vi "Test add points.vi"() -> ()   [LabVIEW 2019]
uses:
  Ctrl/cmd_common.ctl
panel:
  in  "tap":enum32{"Main", "Data"}(tab)
  out "Potential graph":dbl[][](graph)
  in  "Run":bool
  in  "clear":bool
  out "N of obstacles":i32(slide) scale=0.0..20.0
  in  "add obstacle":bool
  in  "Finish":bool
  out "Waypoint":cluster{"add arr":cluster{i32, i32}[]}[](graph)
  in  "global-val":T1={"KP"=5.0, "ETA"=100.0, "AREA_WIDTH"=30.0, "Osc_Det_Len"=3}
  in  "set-val":T2={"start pt"={"x"=0, "y"=10}, "goal pt"={"x"=30, "y"=30}, "grid size"=0.5, "robot radius"=5.0, "obstacles"=[{"x"=15, "y"=25}, {"x"=5, "y"=15}, {"x"=20, "y"=26}, {"x"=25, "y"=25}]}
  in  "add arr":cluster{i32, i32}[](array[cluster])
  out "add point":cluster{i32, i32}
  # "Made by Ybbaek"
  # "Potential Field Simulation"
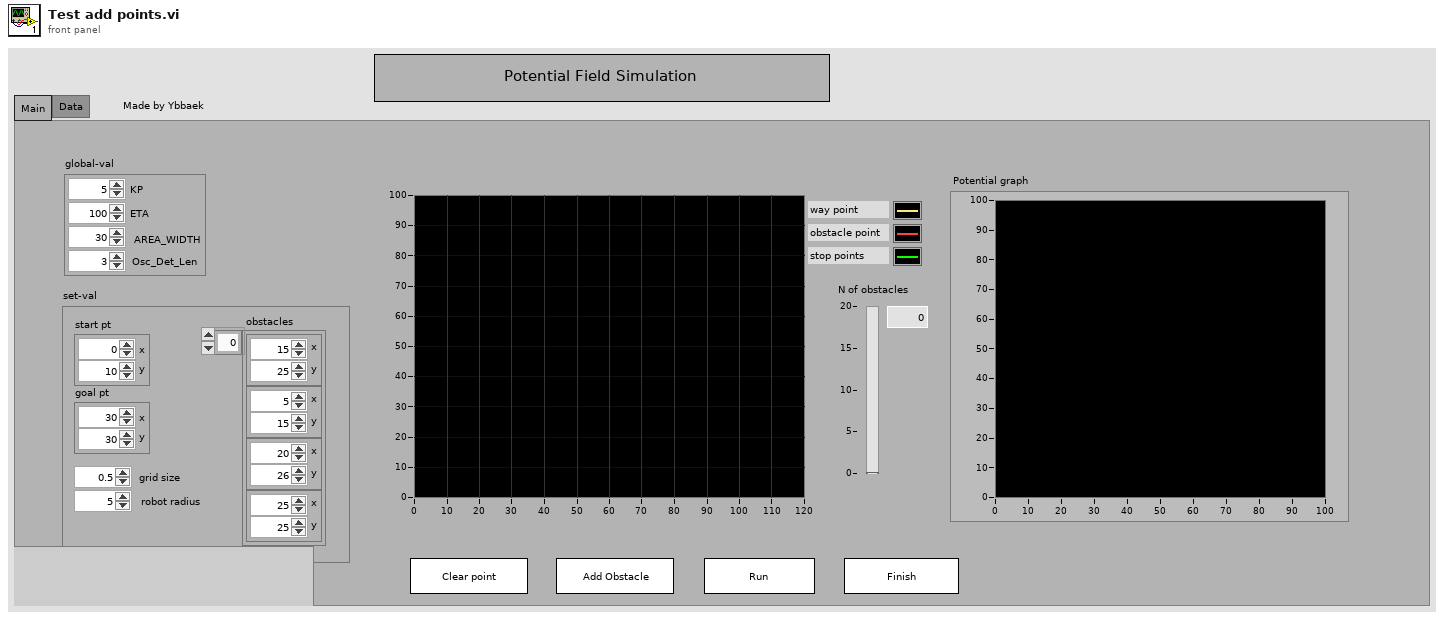
[diagram p1: front panel]
types:
  T1 = cluster{"KP":dbl, "ETA":dbl, "AREA_WIDTH":dbl, "Osc_Det_Len":u32}
  T2 = cluster{"start pt":cluster{"x":i32, "y":i32}, "goal pt":cluster{"x":i32, "y":i32}, "grid size":dbl, "robot radius":dbl, "obstacles":cluster{"x":i32, "y":i32}[]}
  T3 = typedef "cmd_common.ctl" = enum16{"read", "write"}
  T4 = typedef "LVPoint32TypeDef.ctl" = cluster{"Horizontal":i32, "Vertical":i32}
  T5 = typedef "LVRectTypeDef.ctl" = cluster{"Left":i16, "Top":i16, "Right":i16, "Bottom":i16}
  T6 = typedef "NI_Matrix.lvlib/RealMatrix.ctl" = dbl[][]
  T7 = cluster{"delay":dbl, "d":dbl, "rxy":cluster{"x":dbl, "y":dbl}[], "pmap":T6}
  T8 = cluster{"start pt":cluster{"x":i32, "y":dbl}, "goal pt":cluster{"x":dbl, "y":dbl}, "grid size":dbl, "robot radius":dbl, "obstacles":cluster{"x":i32, "y":i32}[]}
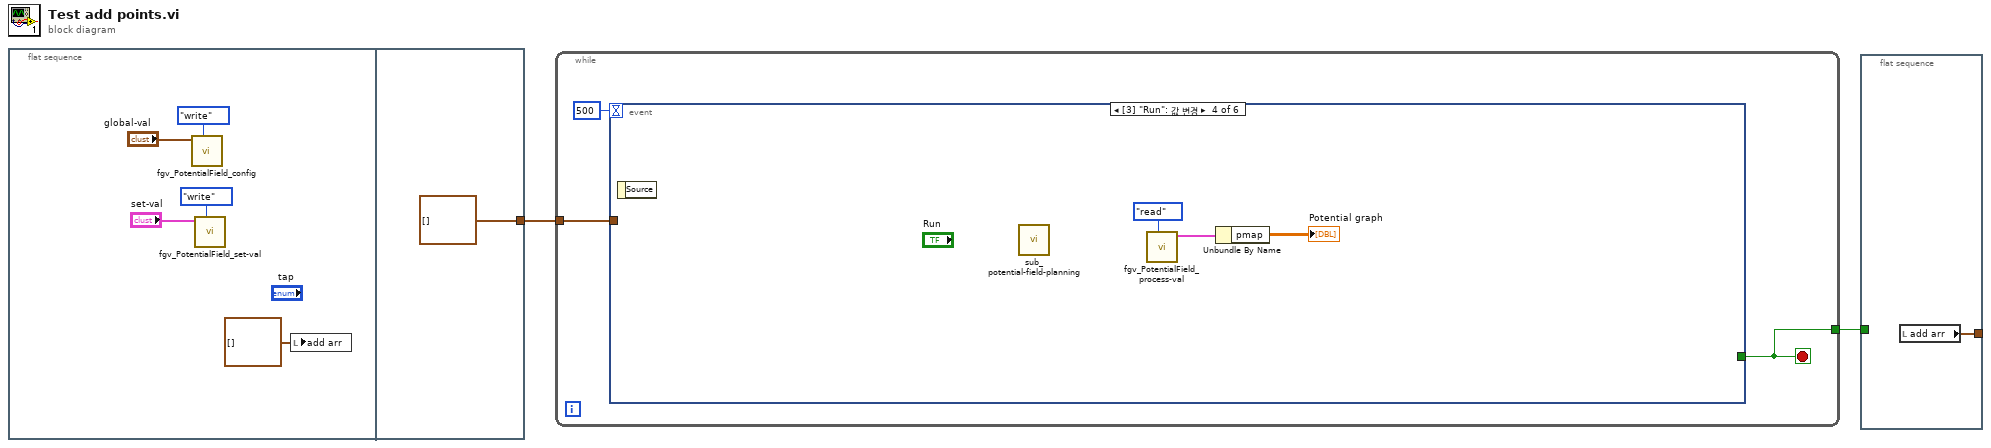
[diagram p0: block diagram]
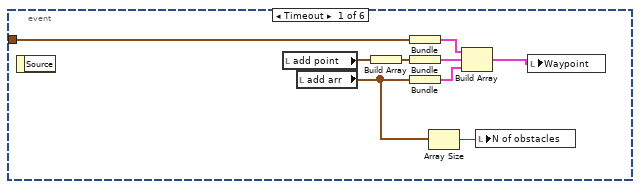
[diagram p2: hidden frame]
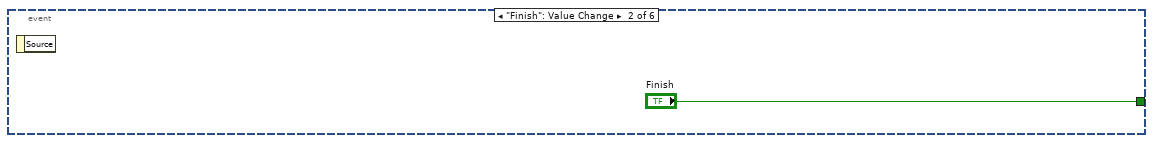
[diagram p3: hidden frame]
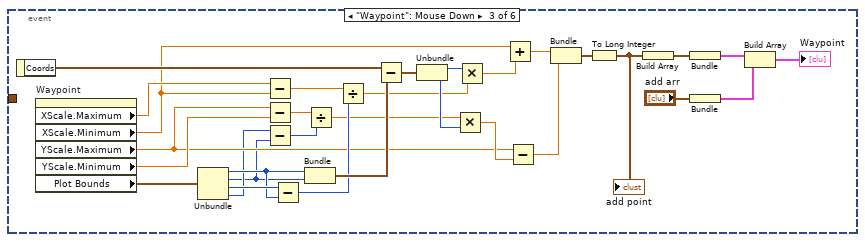
[diagram p4: hidden frame]
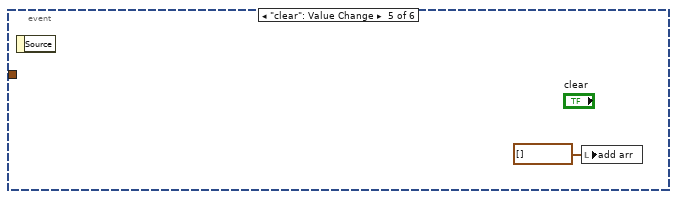
[diagram p5: hidden frame]
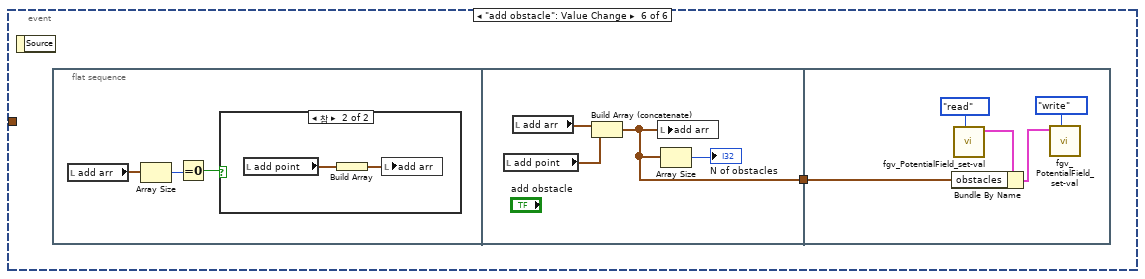
[diagram p6: hidden frame]
diagram:
  n1 = flat-sequence {
    tunnel: [cluster{"X":i32, "Y":i32}[] []] -> w1
    frame #0 {
      n2 = call "fgv_PotentialField_config.vi"("cmd"=cmd_common."write", "pf-val"="global-val") -> ()  [unwired: 9 in, 1 out]
      n3 = call "fgv_PotentialField_set-val.vi"("cmd"=cmd_common."write", "set-val"="set-val") -> ()  [unwired: 9 in, 1 out]
      n4 = local write "add arr"(cluster{i32, i32}[] [] ("add arr")) -> ()
    }
    frame #1 {
    }
  }
  n5 = while {
    tunnel: [w11] -> w2
    tunnel: w1 -> [w10]
    stop <- w11 stop-if-true
    n6 = event shown="[3] \"Run\": 값 변경" {
      selector: _ -> [_ _ _ _ _ _]
      dyn-events: _ -> [_ _ _ _ _ _]
      timeout: 500 -> [_ _ _ _ _ _]
      tunnel: [_ "Finish" _ _ _ _] -> w11
      tunnel: w10 -> [w14 _ _ _ _ _]
      event Timeout {
        n7 = event-data() -> ()  [unwired: 1 in, 1 out]
        n8 = local read "add point"() -> (w19:cluster{i32, i32})
        n9 = local read "add arr"() -> (w12:cluster{i32, i32}[])
        n10 = Build Array(w19) -> (w20:cluster{i32, i32}[])
        n11 = Bundle(w14) -> (w15:cluster{cluster{"X":i32, "Y":i32}[]})  [unwired: 1 in]
        n12 = Bundle(w20) -> (w18:cluster{cluster{i32, i32}[]})  [unwired: 1 in]
        n13 = Bundle("add arr"=w12) -> (w17:cluster{"add arr":cluster{i32, i32}[]})  [unwired: 1 in]
        n14 = Array Size(array=w12) -> (size(s)=w13:i32)
        n15 = Build Array(w15, w18, w17) -> (w16:cluster{"add arr":cluster{"X":i32, "Y":i32}[]}[])
        n16 = local write "N of obstacles"(w13) -> ()
        n17 = local write "Waypoint"(w16) -> ()
      }
      event "Finish": Value Change {
        n18 = event-data() -> ()  [unwired: 1 in, 1 out]
      }
      event "Waypoint": Mouse Down {
        n19 = event-data() -> ("Coords"=w51:T4)  [unwired: 1 in]
        n20 = property on="Waypoint" class="XYGraph (엄격한)"() -> ("XScale.Maximum"=w47:dbl, "XScale.Minimum"=w39:dbl, "YScale.Maximum"=w31:dbl, "YScale.Minimum"=w34:dbl, "Plot Bounds"=w52:T5)  [unwired: 2 in, 2 out]
        n21 = Unbundle(w52) -> ("Left"=w43:i16, "Top"=w29:i16, "Right"=w44:i16, "Bottom"=w30:i16)
        n22 = Subtract(x=w47, y=w39) -> (x-y=w42:dbl)
        n23 = Subtract(x=w31, y=w34) -> (x-y=w37:dbl)
        n24 = Subtract(x=w30, y=w29) -> (x-y=w36:i16)
        n25 = Subtract(x=w44, y=w43) -> (x-y=w41:i16)
        n26 = Bundle("Left"=w43, "Top"=w29) -> (w50:cluster{"Left":i16, "Top":i16})  [unwired: 1 in]
        n27 = Divide(x=w37, y=w36) -> (x/y=w35:dbl)
        n28 = Divide(x=w42, y=w41) -> (x/y=w24:dbl)
        n29 = Subtract(x=w51, y=w50) -> (x-y=w46:T4)
        n30 = Unbundle(w46) -> ("Horizontal"=w25:i32, "Vertical"=w45:i32)
        n31 = Multiply(x=w35, y=w45) -> (x*y=w33:dbl)
        n32 = Multiply(x=w25, y=w24) -> (x*y=w40:dbl)
        n33 = Add(x=w39, y=w40) -> (x+y=w38:dbl)
        n34 = Subtract(x=w31, y=w33) -> (x-y=w32:dbl)
        n35 = Bundle(w38, w32) -> (w23:cluster{dbl, dbl})  [unwired: 1 in]
        n36 = To Long Integer(number=w23) -> (32bit integer=w22:cluster{i32, i32})
        "add point" <- w22
        n37 = Build Array(w22) -> (w48:cluster{i32, i32}[])
        n38 = Bundle(w48) -> (w49:cluster{cluster{i32, i32}[]})  [unwired: 1 in]
        n39 = Bundle("add arr"="add arr") -> (w27:cluster{"add arr":cluster{i32, i32}[]})  [unwired: 1 in]
        n40 = Build Array(w49, w27) -> (→"Waypoint":cluster{"add arr":cluster{i32, i32}[]}[])
      }
      event "Run": Value Change {
        n41 = event-data() -> ()  [unwired: 1 in, 1 out]
        n42 = call "sub_potential-field-planning.vi"() -> ()  [unwired: 12 in]
        n43 = call "fgv_PotentialField_process-val.vi"("cmd"=cmd_common."read") -> ("prcess val out"=w54:T7)  [unwired: 10 in]
        n44 = Unbundle By Name(w54) -> ("pmap"=→"Potential graph":T6)
      }
      event "clear": Value Change {
        n45 = event-data() -> ()  [unwired: 1 in, 1 out]
        n46 = local write "add arr"(cluster{dbl, dbl}[] [] ("add arr")) -> ()
      }
      event "add obstacle": Value Change {
        n47 = event-data() -> ()  [unwired: 1 in, 1 out]
        n48 = flat-sequence {
          tunnel: [w63] -> w57
          tunnel: w57 -> [w67]
          frame #0 {
            n49 = local read "add arr"() -> (w60:cluster{i32, i32}[])
            n50 = Array Size(array=w60) -> (size(s)=w59:i32)
            n51 = Equal To 0?(x=w59) -> (x = 0?=w58:bool)
            n52 = case shown="참" w58 {
              frame False {
              }
              frame True {
                n53 = local read "add point"() -> (w62:cluster{i32, i32})
                n54 = Build Array(w62) -> (w61:cluster{i32, i32}[])
                n55 = local write "add arr"(w61) -> ()
              }
            }
          }
          frame #1 {
            n56 = local read "add point"() -> (w65:cluster{i32, i32})
            n57 = local read "add arr"() -> (w66:cluster{i32, i32}[])
            n58 = Build Array (concatenate)(w66, w65) -> (w63:cluster{i32, i32}[])
            n59 = local write "add arr"(w63) -> ()
            n60 = Array Size(array=w63) -> (size(s)=→"N of obstacles":i32)
          }
          frame #2 {
            n61 = call "fgv_PotentialField_set-val.vi"("cmd"=cmd_common."read") -> ("set-val out"=w69:T8)  [unwired: 10 in]
            n62 = Bundle By Name(cluster=w69, "obstacles"=w67) -> (w68:T8)
            n63 = call "fgv_PotentialField_set-val.vi"("cmd"=cmd_common."write", "set-val"=w68) -> ()  [unwired: 9 in, 1 out]
          }
        }
      }
    }
  }
  n64 = flat-sequence {
    tunnel: w2 -> [_]
    tunnel: [w72] -> _
    frame #0 {
      n65 = local read "add arr"() -> (w72:cluster{i32, i32}[])
    }
  }
